vi "Data Logger.vi"(7 "Action":enum16{"Init", "Save", "Close"}(ring), 8 "error in":errorcluster, 10 "Log File":path, 11 "Data Array In":T1[](array[typedef])) -> (0 "error out":errorcluster)   [LabVIEW 2018]
uses:
  Vacuum Output.ctl
  Main Globals.vi
  Lib/Utilities.lvlib
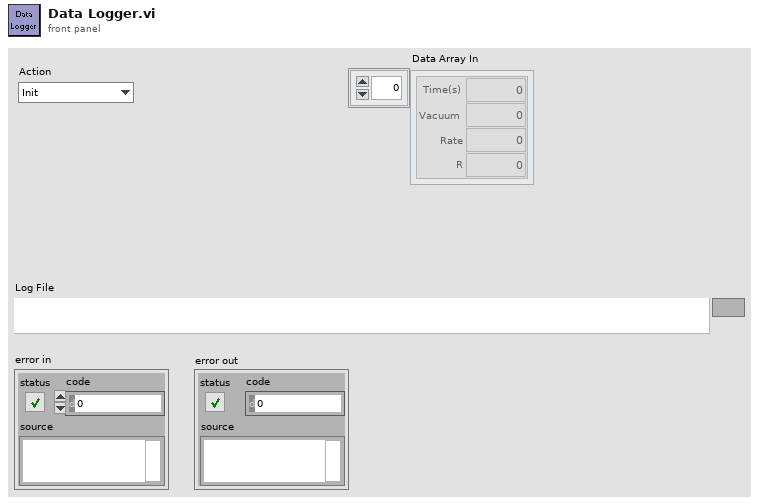
[diagram p1: front panel]
types:
  T1 = typedef "Vacuum Output.ctl" = cluster{"Time(s)":dbl, "Vacuum":dbl, "Rate":dbl, "R":dbl}
  T2 = enum16{"open", "replace", "create", "open or create", "replace or create", "replace or create with confirmation"}
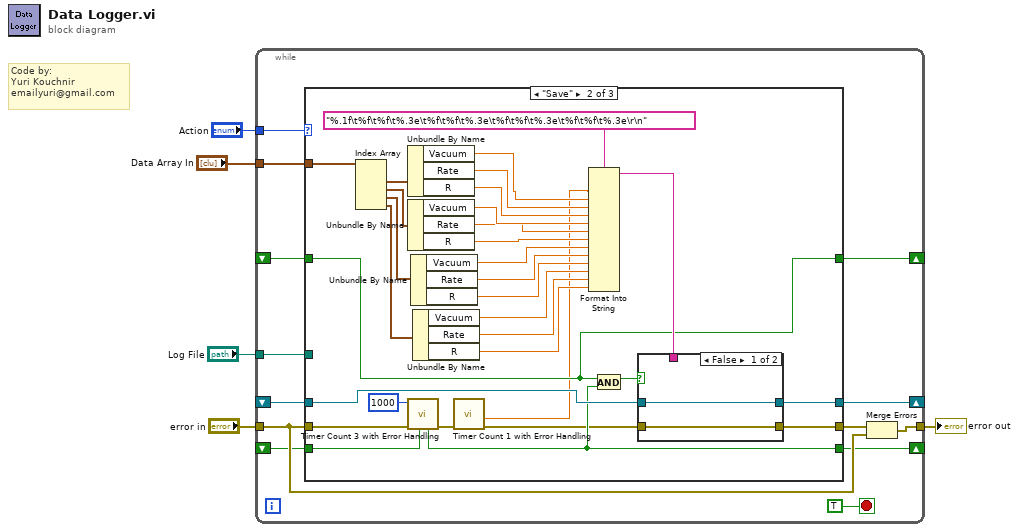
[diagram p0: block diagram]
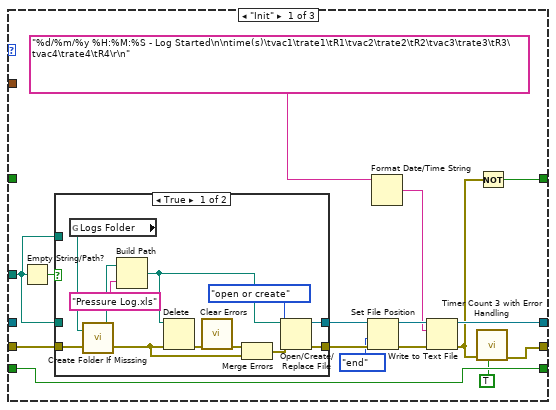
[diagram p2: hidden frame]
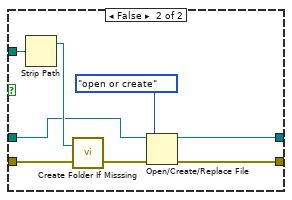
[diagram p3: hidden frame]
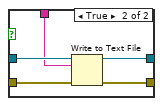
[diagram p4: hidden frame]
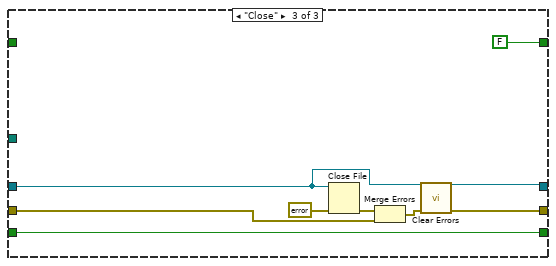
[diagram p5: hidden frame]
diagram:
  # "Code by:\nYuri Kouchnir\nemailyuri@gmail.com"
  n1 = while {
    tunnel: "error in" -> [w11]
    tunnel: [w12] -> w4
    tunnel: "Action" -> [w17]
    tunnel: "Log File" -> [w16]
    shift-right: [w14] -> _
    shift-left: _ -> [w13]
    tunnel: "Data Array In" -> [w10]
    shift-right: [w9] -> _
    shift-left: _ -> [w8]
    shift-right: [w7] -> _
    shift-left: _ -> [w6]
    stop <- TRUE stop-if-true
    n2 = case shown="\"Save\"" w17 {
      tunnel: w16 -> [w33 _ _]
      tunnel: [w20 w84 w98] -> w15
      tunnel: [w27 w85 w95] -> w14
      tunnel: w13 -> [_ w62 w95]
      tunnel: w11 -> [w24 w64 w94]
      tunnel: w10 -> [_ w83 _]
      tunnel: [w23 w65 FALSE ("Record Data")] -> w9
      tunnel: w8 -> [_ w65 _]
      tunnel: [w22 w61 w93] -> w7
      tunnel: w6 -> [w22 w60 w93]
      frame "Init" {
        n3 = Empty String/Path?(string/path=w33) -> (empty?=w34:bool)
        n4 = case shown="True" w34 {
          tunnel: w24 -> [w40 w47]
          tunnel: [w42 w53] -> w32
          tunnel: w33 -> [_ w51]
          tunnel: w33 -> [_ w49]
          tunnel: [w41 w50] -> w31
          frame True {
            n5 = global read "Main Globals.vi" "Logs Folder"() -> (w46:path)
            n6 = call "Create Folder If Misssing.vi"("error in"=w40, "Path In"=w46) -> ("error out"=w37:errorcluster, "Path Out"=w45:path)
            n7 = Build Path(base path=w45, name or relative path="Pressure Log.xls") -> (appended path=w35:path)
            n8 = Delete(path (use dialog)=w35, error in=w37) -> (error out=w39:errorcluster)  [unwired: 3 in, 2 out]
            n9 = call <vilib>:"Clear Errors.vi"("error in (no error)"=w39) -> ("error out"=w36:errorcluster)  [unwired: 5 in, 1 out]
            n10 = Merge Errors(w36, w37) -> (w38:errorcluster)
            n11 = Open/Create/Replace File(file path (use dialog)=w35, error in=w38, operation (0:open)=T2."open or create") -> (refnum out=w41:refnum<file>, error out=w42:errorcluster)  [unwired: 3 in, 1 out]
          }
          frame False {
            n12 = Strip Path(path=w51) -> (stripped path=w52:path)  [unwired: 1 out]
            n13 = call "Create Folder If Misssing.vi"("error in"=w47, "Path In"=w52) -> ("error out"=w48:errorcluster)  [unwired: 1 out]
            n14 = Open/Create/Replace File(file path (use dialog)=w49, error in=w48, operation (0:open)=T2."open or create") -> (refnum out=w50:refnum<file>, error out=w53:errorcluster)  [unwired: 3 in, 1 out]
          }
        }
        n15 = Set File Position(refnum=w31, from (0:start)=enum16{"start", "end", "current"}."end", error in=w32) -> (refnum out=w29:refnum<file>, error out=w26:errorcluster)  [unwired: 1 in]
        n16 = Format Date/Time String(time format string (%c)="%d/%m/%y %H:%M:%S - Log Started\n\ntime(s)\tvac1\trate1\tR1\tvac2\trate2\tR2\tvac3\trate3\tR3\tvac4\trate4\tR4\r\n") -> (date/time string=w25:string)  [unwired: 2 in]
        n17 = Write to Text File(file (use dialog)=w29, text=w25, error in=w26) -> (refnum out=w27:refnum<file>, error out=w21:errorcluster)  [unwired: 1 in, 1 out]
        n18 = call "Timer Count 3 with Error Handling.vi"("Reset"=TRUE, "error in (no error)"=w21) -> ("error out"=w20:errorcluster)  [unwired: 5 in, 4 out]
        n19 = Not(x=w21) -> (.not. x?=w23:bool)
      }
      frame "Save" {
        n20 = Index Array(array=w83) -> (element #1=w82:T1, element #2=w81:T1, element #3=w80:T1, element #4=w79:T1)  [unwired: 4 in]
        n21 = Unbundle By Name(w82) -> ("Vacuum"=w56:dbl, "Rate"=w78:dbl, "R"=w77:dbl)
        n22 = Unbundle By Name(w81) -> ("Vacuum"=w76:dbl, "Rate"=w75:dbl, "R"=w74:dbl)
        n23 = call "Timer Count 3 with Error Handling.vi"("Reset"=w60, "error in (no error)"=w64, "Timeout (ms)"=u32 1000) -> ("error out"=w58:errorcluster, "Timer Elapsed?"=w61:bool)  [unwired: 4 in, 3 out]
        n24 = Unbundle By Name(w80) -> ("Vacuum"=w73:dbl, "Rate"=w72:dbl, "R"=w71:dbl)
        n25 = Unbundle By Name(w79) -> ("Vacuum"=w70:dbl, "Rate"=w69:dbl, "R"=w66:dbl)
        n26 = call "Timer Count 1 with Error Handling.vi"("error in (no error)"=w58) -> ("error out"=w57:errorcluster, "Elapsed Time(s)"=w55:dbl)  [unwired: 7 in, 2 out]
        n27 = Format Into String(format string="%.1f\t%f\t%f\t%.3e\t%f\t%f\t%.3e\t%f\t%f\t%.3e\t%f\t%f\t%.3e\r\n", w55, w56, w78, w77, w76, w75, w74, w73, w72, w71, w70, w69, w66) -> (resulting string=w67:string)  [unwired: 2 in, 1 out]
        n28 = And(x=w65, y=w61) -> (x .and. y?=w63:bool)
        n29 = case shown="False" w63 {
          tunnel: w62 -> [w87 w92]
          tunnel: [w87 w91] -> w85
          tunnel: [w86 w90] -> w84
          tunnel: w57 -> [w86 w89]
          tunnel: w67 -> [_ w88]
          frame False {
          }
          frame True {
            n30 = Write to Text File(file (use dialog)=w92, text=w88, error in=w89) -> (refnum out=w91:refnum<file>, error out=w90:errorcluster)  [unwired: 1 in, 1 out]
          }
        }
      }
      frame "Close" {
        n31 = Close File(refnum=w95, error in=errorcluster {"status"=FALSE, "code"=0, "source"=""}) -> (error out=w100:errorcluster)  [unwired: 1 out]
        n32 = Merge Errors(w100, w94) -> (w97:errorcluster)
        n33 = call <vilib>:"Clear Errors.vi"("error in (no error)"=w97) -> ("error out"=w98:errorcluster)  [unwired: 5 in, 1 out]
      }
    }
    n34 = Merge Errors(w15, w11) -> (w12:errorcluster)
  }
  "error out" <- w4
